vi "scale.vi"(8 "error in (no error)":errorcluster, 9 "y":i32=1, 10 "x":i32=1, 11 "Image in":refnum<class "Image.lvclass">) -> (0 "error out":errorcluster, 3 "Image out":refnum<class "Image.lvclass">)   [LabVIEW 2010, in "Image.lvclass"]
uses:
  Image.lvclass
  storage_mode.ctl
  ErrorController/ErrorController/class_data.vi
  <vilib>/vision/NI_Vision_Development_Module.lvlib
  ErrorController/ErrorController/ErrorController.lvclass
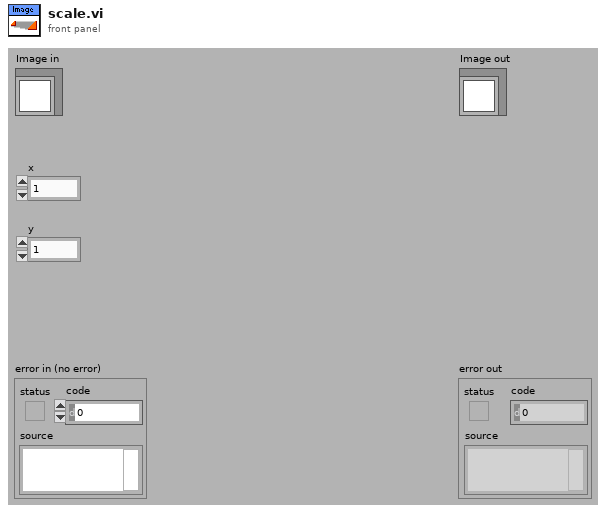
[diagram p1: front panel]
types:
  T1 = typedef "Image.lvclass/storage_mode.ctl" = enum16{"RAM", "disk"}
  T2 = typedef "IMAQ Image.ctl" = refnum<image>
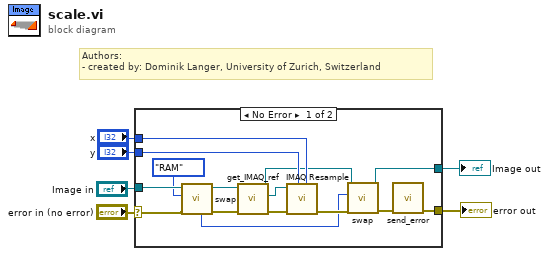
[diagram p0: block diagram]
diagram:
  # "Authors: \n- created by: Dominik Langer, University of Zurich, Switzerland"
  n1 = case shown="No Error" "error in (no error)" {
    selector: "error in (no error)" -> [w15 w23]
    tunnel: [w7 w23] -> w5
    tunnel: [w9 w22] -> w3
    tunnel: "Image in" -> [w16 w22]
    tunnel: "x" -> [w18 _]
    tunnel: "y" -> [w19 _]
    frame No Error {
      n2 = call-dynamic "swap.vi"("error in (no error)"=w15, "storage type target"=storage_mode."RAM", "Image in"=w16) -> ("error out"=w17:errorcluster, "Image out"=w11:refnum<class "Image.lvclass">, "previous storage mode"=w13:T1)  [unwired: 6 out]
      n3 = call-dynamic "get_IMAQ_ref.vi"("error in (no error)"=w17, "Image.lvclass in"=w11) -> ("error out"=w21:errorcluster, "Image"=w20:T2, "Image.lvclass out"=w10:refnum<class "Image.lvclass">)  [unwired: 7 out]
      n4 = call "IMAQ Resample"("X Resolution"=w18, "Y Resolution"=w19, "error in (no error)"=w21, "Image Src"=w20) -> ("error out"=w14:errorcluster)  [unwired: 3 in, 4 out]
      n5 = call-dynamic "swap.vi"("error in (no error)"=w14, "storage type target"=w13, "Image in"=w10) -> ("error out"=w8:errorcluster, "Image out"=w9:refnum<class "Image.lvclass">)  [unwired: 7 out]
      n6 = call "send_error.vi"("error in (no error)"=w8) -> ("error out"=w7:errorcluster)  [unwired: 10 in]
    }
    frame Error {
    }
  }
  "error out" <- w5
  "Image out" <- w3
